vi "R1FourHeadISE.vi"() -> ()   [LabVIEW 2016]
uses:
  Controls/Tri State Control.ctl
  <vilib>/Utility/file.llb/Write Delimited Spreadsheet (string).vi
  <vilib>/Utility/file.llb/Write Delimited Spreadsheet (DBL).vi
panel:
  out "output array":dbl[][](array[numeric])
  out "Plots":cluster{dbl, dbl, dbl}(graph)
  in  "Array 2":string[][](array[string])
  out "Equilibrium?":bool[][](array[boolean])=[[FALSE, TRUE, FALSE, FALSE, TRUE, TRUE]]
  in  "Stabilzation \nCriterion (mV/min)":dbl=0.4
  in  "Differential Window Size (sec)":i64=5
  in  "error in":errorcluster
  out "error out":errorcluster={"status"=TRUE, "code"=7, "source"=""}
  in  "File Name:":string="ISE_Measurements"
  out "new file path (Not A Path if cancelled)":path
  in  "stop":bool
  out "Saving?":bool=TRUE
  out "File Headers":string[][](array[string])=[["Unix Time Code - 8hrs", "M6AI2", "M6AI4", "M6AI6", "M6AI16", "M6AI18", "M6AI20"], ["Unix Time Code - 8hrs", "NH4+", "Ca2+", "K+", "Na+", "Cl-", "NO3-"]]
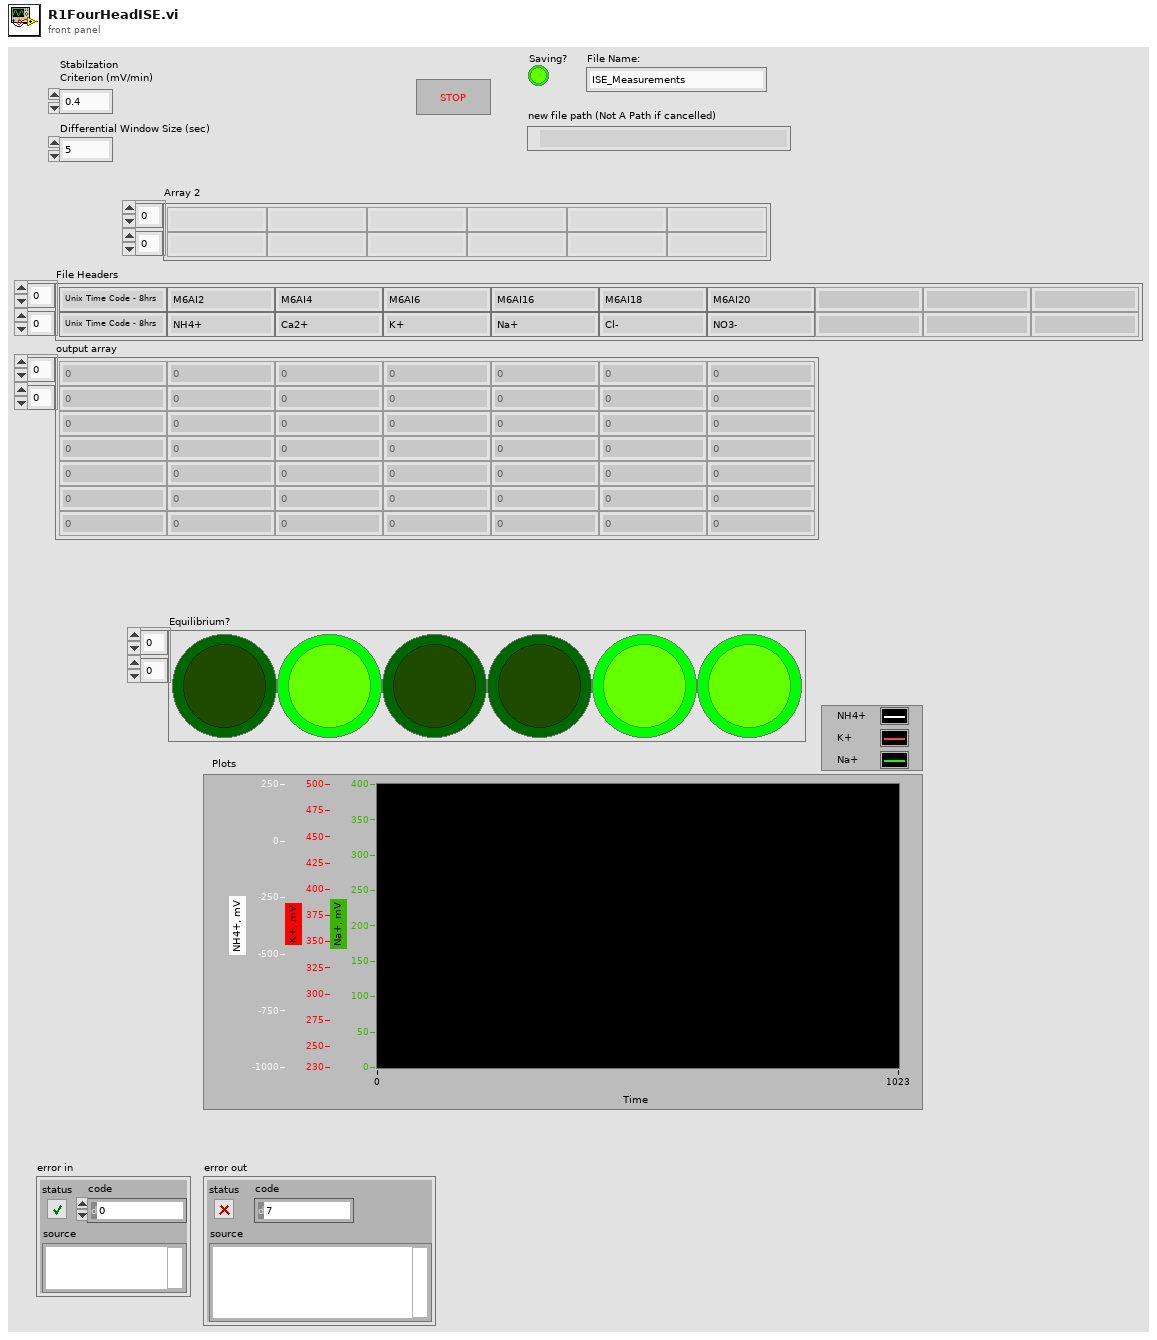
[diagram p1: front panel]
types:
  T1 = typedef "Tri State Control.ctl" = u16
  T2 = cluster{"Raw Value":dbl, "Corrected Value":dbl, "Signal, mV":dbl, "Equilibrium Approach, mV/min":dbl, "Steady State?":T1}
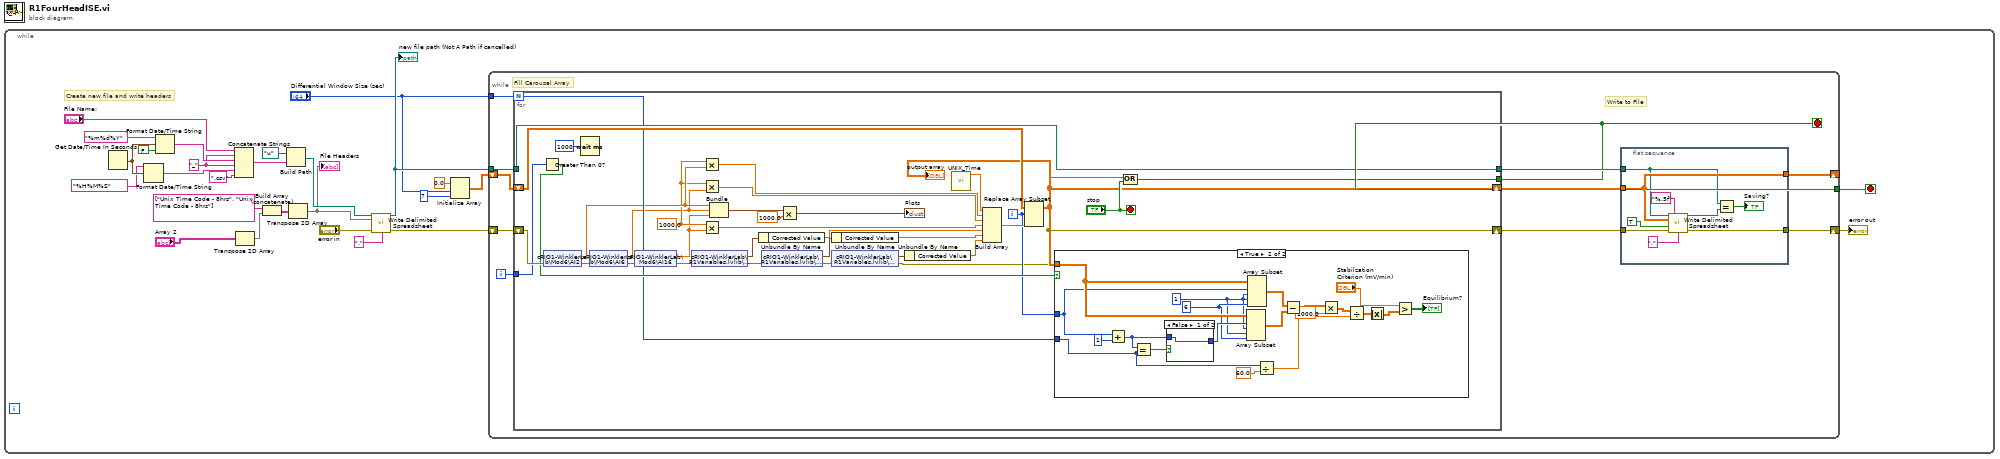
[diagram p0: block diagram]
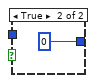
[diagram p3: hidden frame]
diagram:
  n1 = while {
    stop <- w3 stop-if-true
    w16 = "_" ("string")
    # "Create new file and write headers"
    n2 = Get Date/Time In Seconds() -> (seconds since 1Jan1904=w21:timestamp)
    n3 = Format Date/Time String(time format string (%c)="%H%M%S", seconds (now)=w21) -> (date/time string=w15:string)  [unwired: 1 in]
    n4 = Format Date/Time String(time format string (%c)="%m%d%Y", seconds (now)=w21, UTC format=FALSE) -> (date/time string=w17:string)
    n5 = Concatenate Strings("File Name:", w16, w17, w16, w15, ".csv" ("string")) -> (w14:string)
    n6 = Transpose 2D Array(2D array="Array 2") -> (transposed array=w9:string[][])
    n7 = Build Array (concatenate)(string[] ["Unix Time Code - 8hrs", "Unix Time Code - 8hrs"], w9) -> (w10:string[][])
    n8 = Build Path(base path=path "u:/" ("Save to:"), name or relative path=w14) -> (appended path=w23:path)
    n9 = Transpose 2D Array(2D array=w10) -> (transposed array=w8:string[][])
    "File Headers" <- w8
    n10 = call-poly <vilib>:"Write Delimited Spreadsheet.vi"("file path (dialog if empty)"=w23, "2D data"=w8, "error in (no error)"="error in", "delimiter (\\t)"="," ("delimiter (\\t)")) -> ("new file path (Not A Path if cancelled)"=w27:path, "error out"=w26:errorcluster)  [unwired: 10 in]
    "new file path (Not A Path if cancelled)" <- w27
    n11 = Initialize Array(0.0 ("element"), "Differential Window Size (sec)", 7 ("dimension size")) -> (w4:dbl[][])
    n12 = while {
      tunnel: w27 -> [w38]
      shift-right: [w34] -> w11
      shift-left: w26 -> [w37]
      tunnel: "Differential Window Size (sec)" -> [w33]
      shift-right: [w31] -> _
      shift-left: w4 -> [w30]
      tunnel: [w29] -> w3
      i -> [w28]
      stop <- w29 stop-if-true
      # "Fill Carousel Array"
      # "Write to File"
      n13 = for {
        N: w33 -> [w72]
        tunnel: w38 -> [w79]
        tunnel: [w75] -> w29
        shift-right: [w61] -> w35
        shift-left: w37 -> [w81]
        tunnel: [w79] -> w32
        shift-right: [w74] -> w36
        shift-left: w30 -> [w78]
        tunnel: w28 -> [w71]
        i -> [w70]
        stop <- "stop" stop-if-true
        w54 = 1000.0 ("y")
        n14 = Greater Than 0?(x=w71) -> (x > 0?=w73:bool)
        n15 = shared-variable "cRIO1-WinklerLab\\Mod6\\AI2"(error in=w81) -> (w57:dbl, error out=w50:errorcluster)
        n16 = Wait (ms)(milliseconds to wait=u32 1000) -> ()  [unwired: 1 out]
        n17 = shared-variable "cRIO1-WinklerLab\\Mod6\\AI6"(error in=w50) -> (w51:dbl, error out=w49:errorcluster)
        n18 = shared-variable "cRIO1-WinklerLab\\Mod6\\AI16"(error in=w49) -> (w52:dbl, error out=w48:errorcluster)
        n19 = shared-variable "cRIO1-WinklerLab\\R1Variables.lvlib\\R1ISEVariables.lvlib\\R1_K_ISE"(error in=w48) -> (w69:T2, error out=w63:errorcluster)
        n20 = Multiply(x=w54, y=w57) -> (x*y=w56:dbl)
        n21 = Multiply(x=w54, y=w51) -> (x*y=w55:dbl)
        n22 = Multiply(x=w54, y=w52) -> (x*y=w53:dbl)
        n23 = Bundle(w57, w51, w52) -> (w59:cluster{dbl, dbl, dbl})  [unwired: 1 in]
        n24 = Unbundle By Name(w69) -> ("Corrected Value"=w66:dbl)
        n25 = shared-variable "cRIO1-WinklerLab\\R1Variables.lvlib\\R1ISEVariables.lvlib\\R1_Na_ISE"(error in=w63) -> (w67:T2, error out=w62:errorcluster)
        n26 = Multiply(x=w59, y=1000.0) -> (x*y=→"Plots":cluster{dbl, dbl, dbl})
        n27 = Unbundle By Name(w67) -> ("Corrected Value"=w65:dbl)
        n28 = shared-variable "cRIO1-WinklerLab\\R1Variables.lvlib\\R1ISEVariables.lvlib\\R1_NH4_ISE"(error in=w62) -> (w68:T2, error out=w61:errorcluster)
        n29 = Unbundle By Name(w68) -> ("Corrected Value"=w64:dbl)
        n30 = call "UNIX_Time.vi"() -> ("Unix time"=w82:dbl)  [unwired: 10 in, 1 out]
        n31 = Build Array(w82, w56, w55, w53, w66, w65, w64) -> (w77:dbl[])
        n32 = Replace Array Subset(array=w78, new element=w77, index (row)=w70) -> (w74:dbl[][])  [unwired: 1 in]
        "output array" <- w74
        n33 = case shown="True" w73 {
          tunnel: w74 -> [_ w102]
          tunnel: w70 -> [_ w101]
          tunnel: w72 -> [_ w91]
          frame False {
          }
          frame True {
            w96 = 6 ("length")
            w90 = 1 ("index")
            n34 = Add(x=w101, y=1) -> (x+y=w97:i32)
            n35 = Equal?(x=w97, y=w91) -> (x = y?=w99:bool)
            n36 = case shown="False" w99 {
              tunnel: [w103 0 ("y")] -> w98
              tunnel: w97 -> [w103 _]
              frame False {
              }
              frame True {
              }
            }
            n37 = Array Subset(array=w102, index (row)=w98, length (row)=w90, index (col)=w90, length (col)=w96) -> (w94:dbl[][])
            n38 = Array Subset(array=w102, index (row)=w101, length (row)=w90, index (col)=w90, length (col)=w96) -> (w95:dbl[][])
            n39 = Divide(x=w91, y=60.0) -> (x/y=w93:dbl)
            n40 = Subtract(x=w95, y=w94) -> (x-y=w86:dbl[][])
            n41 = Multiply(x=w86, y=1000.0) -> (x*y=w87:dbl[][])
            n42 = Divide(x=w87, y=w93) -> (x/y=w83:dbl[][])
            n43 = Absolute Value(x=w83) -> (abs(x)=w84:dbl[][])
            n44 = Greater?(x="Stabilzation \nCriterion (mV/min)", y=w84) -> (0:→"Equilibrium?":bool[][])
          }
        }
        n45 = Compound Arithmetic op=OR(w61, "stop") -> (w75:bool)
      }
      n46 = flat-sequence {
        tunnel: w36 -> [w40]
        tunnel: w35 -> [w47]
        tunnel: [w46] -> w34
        tunnel: w32 -> [w39]
        tunnel: [w40] -> w31
        frame #0 {
          n47 = call-poly <vilib>:"Write Delimited Spreadsheet.vi"("file path (dialog if empty)"=w39, "format (%.3f)"="%.5f", "2D data"=w40, "append to file? (new file:F)"=TRUE, "error in (no error)"=w47, "delimiter (\\t)"="," ("delimiter (\\t)")) -> ("new file path (Not A Path if cancelled)"=w44:path, "error out"=w46:errorcluster)  [unwired: 8 in]
          n48 = Equal?(x=w39, y=w44) -> (x = y?=→"Saving?":bool)
        }
      }
    }
    "error out" <- w11
  }
